vi "_API_BINANCE_GET_USDT_FUTURES_allOrders.vi"(0 "BinanceAPI in":refnum<class "BinanceAPI_.lvclass">, 5 "allOrders":T2={"symbol (eg. BTCUSDT)"="", "orderid"=0.0, "startTime"=0, "endTime"=0, "limit"=0, "recvWindow"=5000}, 11 "error in (no error)":errorcluster) -> (4 "BinanceAPI out":refnum<class "BinanceAPI_.lvclass">, 6 "data":T1(array[cluster]), 14 "Dane":string, 15 "error out":errorcluster)   [LabVIEW 2022 SP3, in "BinanceAPI_.lvclass"]
doc: "https://binance-docs.github.io/apidocs/spot/en/#all-orders-user_data"
uses:
  BinanceAPI_.lvclass
  BinanceAPI_.lvclass/BinanceAPI_.ctl
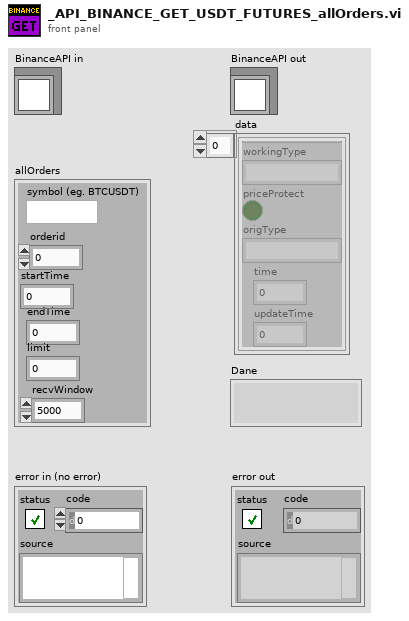
[diagram p1: front panel]
types:
  T1 = cluster{"orderId":dbl, "symbol":string, "status":string, "clientOrderId":string, "price":string, "avgPrice":string, "origQty":string, "executedQty":string, "cumQuote":string, "timeInForce":string, "type":string, "reduceOnly":bool, "closePosition":bool, "side":string, "positionSide":string, "stopPrice":string, "workingType":string, "priceProtect":bool, "origType":string, "time":dbl, "updateTime":dbl}[]
  T2 = cluster{"symbol (eg. BTCUSDT)":string, "orderid":dbl, "startTime":i32, "endTime":i32, "limit":i16, "recvWindow":i32}
  T3 = enum16{"SPOT", "USDT_FUTURES", "COIN_FUTURES", "VANILLA"}
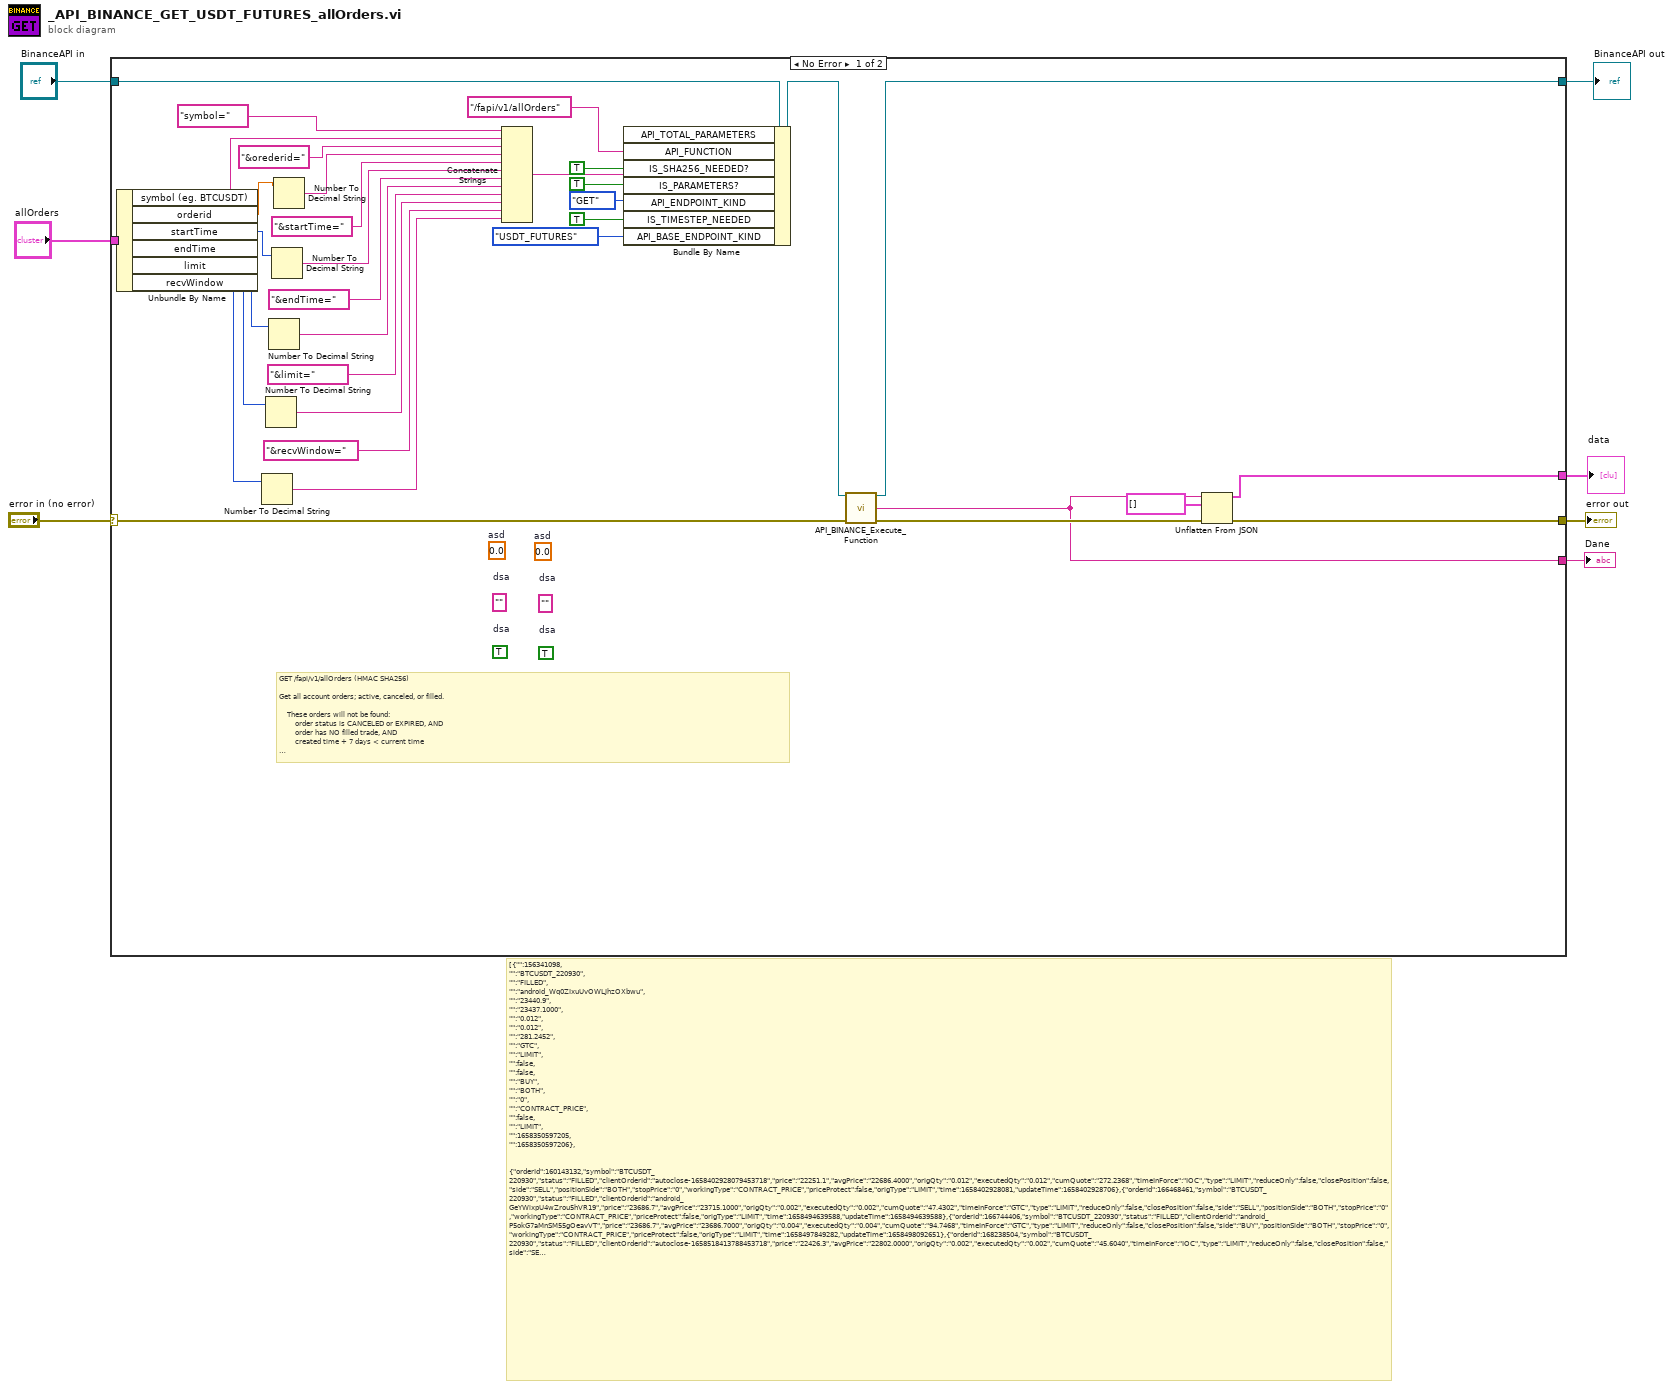
[diagram p0: block diagram]
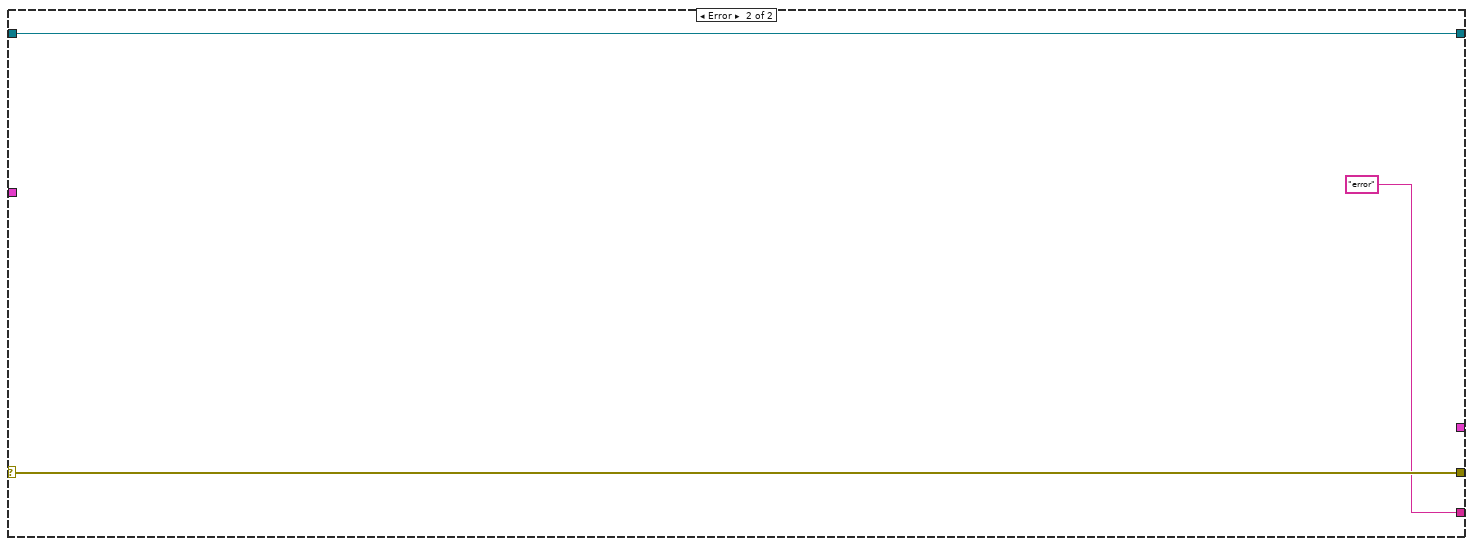
[diagram p2: hidden frame]
diagram:
  # "[{\"\":156341098,\n\"\":\"BTCUSDT_220930\",\n\"\":\"FILLED\",\n\"\":\"android_Wq0ZIxuUvOWLJhzOXbwu\",\n\"\":\"23440.9\",\n\"\":\"23437.1000\",\n\"\":\"0.012\",\n\"\":\"0.012\",\n\"\":\"281.2452\",\n\"\":\"GTC\",\n\"\":\"LIMIT\",\n\"\":false,\n\"\":false,\n\"\":\"BUY\",\n\"\":\"BOTH\",\n\"\":\"0\",\n\"\":\"CONTRACT_PRICE\",\n\"\":false,\n\"\":\"LIMIT\",\n\"\":1658350597205,\n\"\":1658350597206},\n\n\n{\"orderId\":160143132,\"symbol\":\"BTCUSDT_220930\",\"status\":\"FILLED\",\"clientOrderId\":\"autoclose-1658402928079453718\",\"price\":\"22251.1\",\"avgPrice\":\"22686.4000\",\"origQty\":\"0.012\",\"executedQty\":\"0.012\",\"cumQuote\":\"272.2368\",\"timeInForce\":\"IOC\",\"type\":\"LIMIT\",\"reduceOnly\":false,\"closePosition\":false,\"side\":\"SELL\",\"positionSide\":\"BOTH\",\"stopPrice\":\"0\",\"workingType\":\"CONTRACT_PRICE\",\"priceProtect\":false,\"origType\":\"LIMIT\",\"time\":1658402928081,\"updateTime\":1658402928706},{\"orderId\":166468461,\"symbol\":\"BTCUSDT_220930\",\"status\":\"FILLED\",\"clientOrderId\":\"android_GeYWixpU4wZrou5hVR19\",\"price\":\"23686.7\",\"avgPrice\":\"23715.1000\",\"origQty\":\"0.002\",\"executedQty\":\"0.002\",\"cumQuote\":\"47.4302\",\"timeInForce\":\"GTC\",\"type\":\"LIMIT\",\"reduceOnly\":false,\"closePosition\":false,\"side\":\"SELL\",\"positionSide\":\"BOTH\",\"stopPrice\":\"0\",\"workingType\":\"CONTRACT_PRICE\",\"priceProtect\":false,\"origType\":\"LIMIT\",\"time\":1658494639588,\"updateTime\":1658494639588},{\"orderId\":166744406,\"symbol\":\"BTCUSDT_220930\",\"status\":\"FILLED\",\"clientOrderId\":\"android_P5okG7aMnSM55gOeavVT\",\"price\":\"23686.7\",\"avgPrice\":\"23686.7000\",\"origQty\":\"0.004\",\"executedQty\":\"0.004\",\"cumQuote\":\"94.7468\",\"timeInForce\":\"GTC\",\"type\":\"LIMIT\",\"reduceOnly\":false,\"closePosition\":false,\"side\":\"BUY\",\"positionSide\":\"BOTH\",\"stopPrice\":\"0\",\"workingType\":\"CONTRACT_PRICE\",\"priceProtect\":false,\"origType\":\"LIMIT\",\"time\":1658497849282,\"updateTime\":1658498092651},{\"orderId\":168238504,\"symbol\":\"BTCUSDT_220930\",\"status\":\"FILLED\",\"clientOrderId\":\"autoclose-1658518413788453718\",\"price\":\"22426.3\",\"avgPrice\":\"22802.0000\",\"origQty\":\"0.002\",\"executedQty\":\"0.002\",\"cumQuote\":\"45.6040\",\"timeInForce\":\"IOC\",\"type\":\"LIMIT\",\"reduceOnly\":false,\"closePosition\":false,\"side\":\"SELL\",\"positionSide\":\"BOTH\",\"stopPrice\":\"0\",\"workingType\":\"CONTRACT_PRICE\",\"priceProtect\":false,\"origType\":\"LIMIT\",\"time\":1658518413792,\"updateTime\":1658518414311},{\"orderId\":8389765531853875757,\"symbol\":\"ETHUSDT\",\"status\":\"FILLED\",\"clientOrderId\":\"android_deiFAnjZJKz51ke5I1K7\",\"price\":\"1544.48\",\"avgPrice\":\"1544.48000\",\"origQty\":\"0.124\",\"executedQty\":\"0.124\",\"cumQuote\":\"191.51552\",\"timeInForce\":\"GTC\",\"type\":\"LIMIT\",\"reduceOnly\":false,\"closePosition\":false,\"side\":\"BUY\",\"positionSide\":\"BOTH\",\"stopPrice\":\"0\",\"workingType\":\"CONTRACT_PRICE\",\"priceProtect\":false,\"origType\":\"LIMIT\",\"time\":1658745630266,\"updateTime\":1658745638979}]"
  n1 = case shown="No Error" "error in (no error)" {
    selector: "error in (no error)" -> [w31 w44]
    tunnel: [w11 w44] -> w5
    tunnel: [w32 w43] -> w1
    tunnel: "BinanceAPI in" -> [w41 w43]
    tunnel: "allOrders" -> [w28 _]
    tunnel: [w10 "error" ("Dane")] -> w4
    tunnel: [w8 _] -> w3
    frame No Error {
      (unwired) TRUE  # dsa
      (unwired) ""  # dsa
      (unwired) 0.0  # asd
      (unwired) TRUE  # dsa
      (unwired) ""  # dsa
      (unwired) 0.0  # asd
      # "GET /fapi/v1/allOrders (HMAC SHA256)\n\nGet all account orders; active, canceled, or filled.\n\n    These orders will not be found:\n        order status is CANCELED or EXPIRED, AND\n        order has NO filled trade, AND\n        created time + 7 days < current time\n\nWeight: 5\n\nParameters:\nName \tType \tMandatory \tDescription\nsymbol \tSTRING \tYES \t\norderId \tLONG \tNO \t\nstartTime \tLONG \tNO \t\nendTime \tLONG \tNO \t\nlimit \tINT \tNO \tDefault 500; max 1000.\nrecvWindow \tLONG \tNO \t\ntimestamp \tLONG \tYES \t\n\nNotes:\n\n    If orderId is set, it will get orders >= that orderId. Otherwise most recent orders are returned.\n    The query time period must be less then 7 days( default as the recent 7 days)."
      n2 = Unbundle By Name(w28) -> ("symbol (eg. BTCUSDT)"=w27:string, "orderid"=w14:dbl, "startTime"=w26:i32, "endTime"=w25:i32, "limit"=w24:i16, "recvWindow"=w23:i32)
      n3 = Number To Decimal String(number=w23) -> (decimal integer string=w15:string)  [unwired: 1 in]
      n4 = Number To Decimal String(number=w24) -> (decimal integer string=w17:string)  [unwired: 1 in]
      n5 = Number To Decimal String(number=w25) -> (decimal integer string=w19:string)  [unwired: 1 in]
      n6 = Number To Decimal String(number=w26) -> (decimal integer string=w21:string)  [unwired: 1 in]
      n7 = Number To Decimal String(number=w14) -> (decimal integer string=w13:string)  [unwired: 1 in]
      n8 = Concatenate Strings("symbol=", w27, "&orederid=", w13, "&startTime=", w21, "&endTime=", w19, "&limit=", w17, "&recvWindow=", w15) -> (w35:string)
      n9 = Bundle By Name(cluster=w41, "API_TOTAL_PARAMETERS"=w35, "API_FUNCTION"="/fapi/v1/allOrders", "IS_SHA256_NEEDED?"=TRUE, "IS_PARAMETERS?"=TRUE, "API_ENDPOINT_KIND"=enum16{"POST", "DELETE", "GET", "PUT"}."GET", "IS_TIMESTEP_NEEDED"=TRUE, "API_BASE_ENDPOINT_KIND"=T3."USDT_FUTURES") -> (w33:refnum<class "BinanceAPI_.lvclass">)
      n10 = call "API_BINANCE_Execute_Function.vi"("BinanceAPI in"=w33, "error in (no error)"=w31) -> ("BinanceAPI out"=w32:refnum<class "BinanceAPI_.lvclass">, "Body"=w10:string, "error out"=w30:errorcluster)  [unwired: 9 in, 2 out]
      n11 = Unflatten From JSON(JSON string=w10, type and defaults=T1 [], error in (no error)=w30) -> (value=w8:T1, error out=w11:errorcluster)  [unwired: 4 in]
    }
    frame Error {
    }
  }
  "error out" <- w5
  "Dane" <- w4
  "data" <- w3
  "BinanceAPI out" <- w1
